vi "Start DAQ.vi"(8 "error in":errorcluster, 11 "Baseline Mocon \npiD-Tech plus in":refnum<class "Baseline Mocon piD-Tech plus.lvclass">) -> (0 "error out":errorcluster, 3 "Baseline Mocon \npiD-Tech plus out":refnum<class "Baseline Mocon piD-Tech plus.lvclass">)   [LabVIEW 2011, in "Baseline Mocon piD-Tech plus.lvclass"]
uses:
  Baseline Mocon piD-Tech plus.lvclass
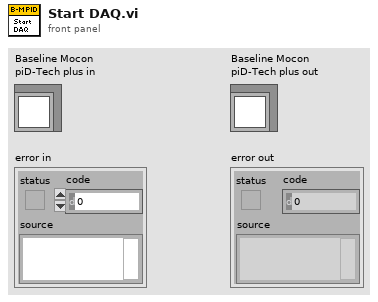
[diagram p1: front panel]
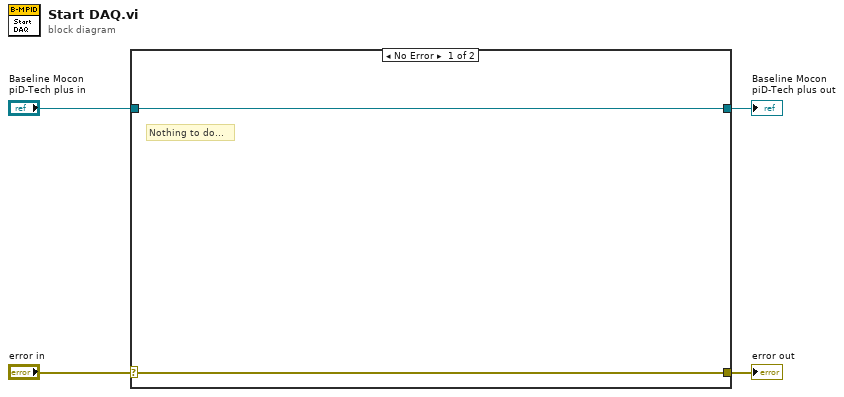
[diagram p0: block diagram]
diagram:
  n1 = case shown="No Error" "error in" {
    selector: "error in" -> [w5 w8]
    tunnel: [w5 w8] -> w3
    tunnel: [w6 w7] -> w1
    tunnel: "Baseline Mocon \npiD-Tech plus in" -> [w6 w7]
    frame No Error {
      # "Nothing to do..."
    }
    frame Error {
    }
  }
  "error out" <- w3
  "Baseline Mocon \npiD-Tech plus out" <- w1
